vi "Read ADC.vi"(8 "error in (no error)":errorcluster, 10 "ADC CH":dbl, 11 "Cypress in":refnum<class "Cypress.lvclass">) -> (0 "error out":errorcluster, 3 "Cypress out":refnum<class "Cypress.lvclass">)   [LabVIEW 2020, in "Cypress.lvclass"]
uses:
  Cypress.lvclass
  a6140e63-044c-432c-b3e2-d1ba8f093480.vi
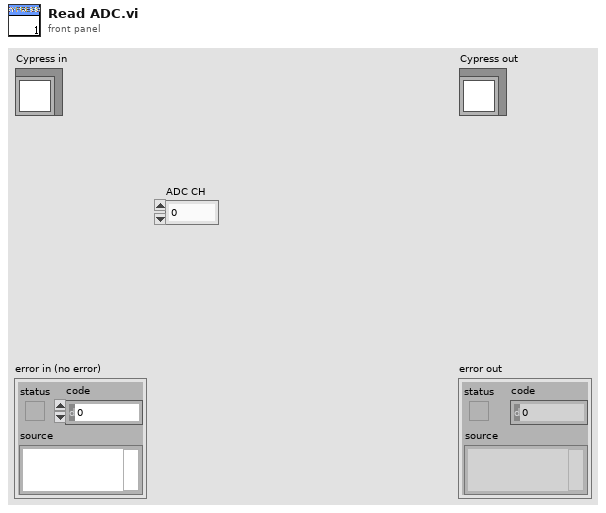
[diagram p1: front panel]
types:
  T1 = typedef "Serial Device.lvclass/serial device brand.ctl" = string
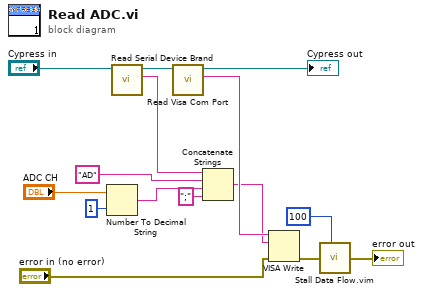
[diagram p0: block diagram]
diagram:
  n1 = Number To Decimal String(number="ADC CH", width (-)=i16 1) -> (decimal integer string=w9:string)
  n2 = call-dynamic "Read Serial Device Brand.vi"("Serial Device in"="Cypress in") -> ("Serial Device Brand"=w11:T1, "Serial Device out"=w15:refnum<class "Cypress.lvclass">)  [unwired: 8 in, 1 out]
  n3 = call-dynamic "Read Visa Com Port.vi"("Serial Device in"=w15) -> ("Visa Com Port"=w3:string, "Serial Device out"=→"Cypress out":refnum<class "Cypress.lvclass">)  [unwired: 8 in, 1 out]
  n4 = Concatenate Strings(w11, "AD" ("string"), w9, ";" ("string")) -> (w2:string)
  n5 = VISA Write(VISA resource name=w3, write buffer=w2, error in (no error)="error in (no error)") -> (error out=w6:errorcluster)  [unwired: 2 out]
  n6 = call "Stall Data Flow.vim"("value in"=w6, "milliseconds to wait"=u32 100) -> ("value out"=→"error out":errorcluster)  [unwired: 1 out]
